vi "longStringToDateTime.vi"(11 "input string":string="2014/01/01 上午 10:00:00") -> (2 "output cluster":T1)   [LabVIEW 2012]
uses:
  <vilib>/Utility/miscctls.llb/LVDateTimeRec.ctl
panel:
  in  "date time rec 2":T1
  in  "date time rec":T1
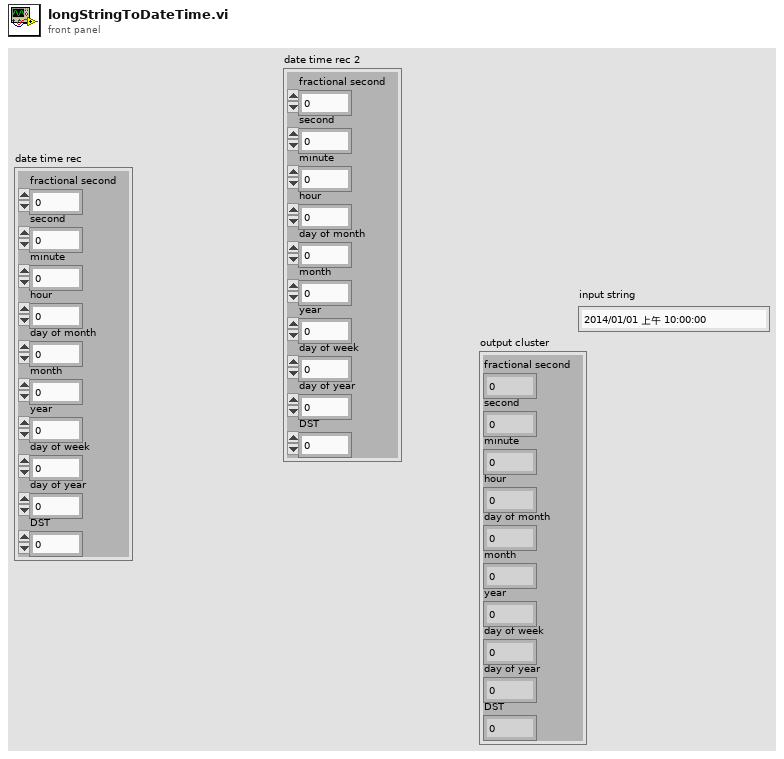
[diagram p1: front panel]
types:
  T1 = typedef "LVDateTimeRec.ctl" = cluster{"fractional second":dbl, "second":i32, "minute":i32, "hour":i32, "day of month":i32, "month":i32, "year":i32, "day of week":i32, "day of year":i32, "DST":i32}
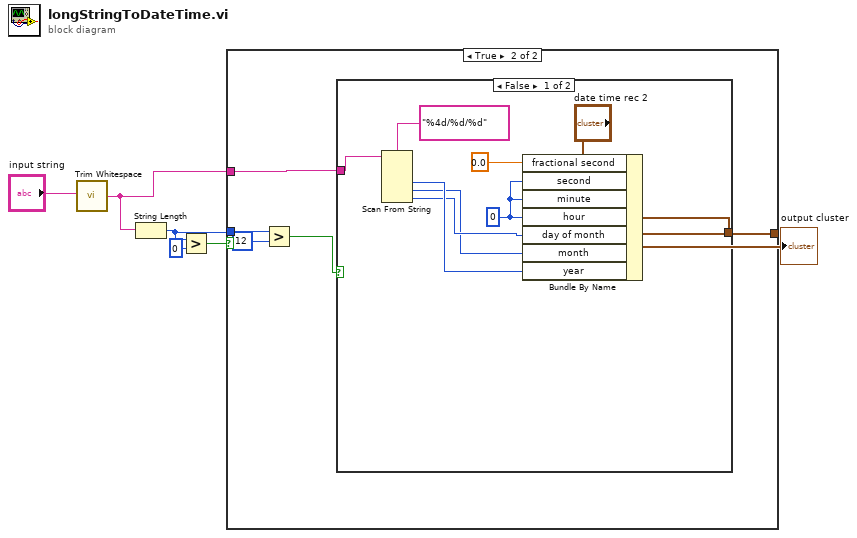
[diagram p0: block diagram]
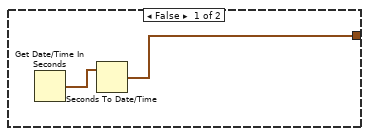
[diagram p2: hidden frame]
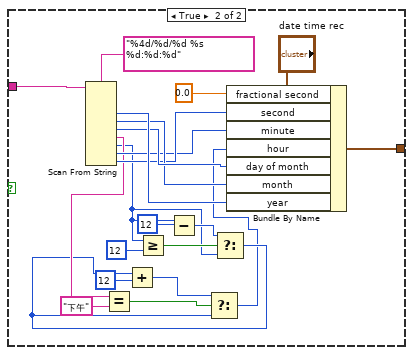
[diagram p3: hidden frame]
diagram:
  n1 = call <vilib>:"Trim Whitespace.vi"("string"="input string") -> ("trimmed string"=w2:string)  [unwired: 1 in]
  n2 = String Length(string=w2) -> (length=w1:i32)
  n3 = Greater?(x=w1, y=0) -> (0:w4:bool)
  n4 = case shown="True" w4 {
    tunnel: [w7 w13] -> w6
    tunnel: w2 -> [_ w12]
    tunnel: w1 -> [_ w11]
    frame False {
      n5 = Get Date/Time In Seconds() -> (seconds since 1Jan1904=w8:timestamp)
      n6 = Seconds To Date/Time(time stamp (now)=w8) -> (date time rec=w7:T1)  [unwired: 1 in]
    }
    frame True {
      n7 = Greater?(x=w11, y=12) -> (0:w9:bool)
      n8 = case shown="False" w9 {
        tunnel: [w14 w36] -> w13
        tunnel: w12 -> [w16 w23]
        frame False {
          w15 = 0 ("hour")
          n9 = Scan From String(format string="%4d/%d/%d", input string=w16) -> (output 1=w19:i32, output 2=w17:i32, output 3=w18:i32)  [unwired: 5 in, 3 out]
          n10 = Bundle By Name(cluster="date time rec 2", "fractional second"=0.0, "second"=w15, "minute"=w15, "hour"=w15, "day of month"=w18, "month"=w17, "year"=w19) -> (w14:T1)
        }
        frame True {
          n11 = Scan From String(format string="%4d/%d/%d %s %d:%d:%d", input string=w23) -> (output 1=w41:i32, output 2=w39:i32, output 3=w40:i32, output 4=w32:string, output 5=w26:i32, output 6=w37:i32, output 7=w38:i32)  [unwired: 9 in, 3 out]
          n12 = Equal?(x=w32, y="下午") -> (x = y?=w30:bool)
          n13 = Greater Or Equal?(x=w26, y=12) -> (x >= y?=w35:bool)
          n14 = Subtract(x=w26, y=12) -> (x-y=w33:i32)
          n15 = Select(t=w33, s=w35, f=w26) -> (s? t:f=w25:i32)
          n16 = Add(x=w25, y=12) -> (x+y=w27:i32)
          n17 = Select(t=w27, s=w30, f=w25) -> (s? t:f=w24:i32)
          n18 = Bundle By Name(cluster="date time rec", "fractional second"=0.0, "second"=w38, "minute"=w37, "hour"=w24, "day of month"=w40, "month"=w39, "year"=w41) -> (w36:T1)
        }
      }
    }
  }
  "output cluster" <- w6
